vi "Main.vi"(8 "error in (no error)":T1) -> (0 "error out":T1)   [LabVIEW 2019, in "GUI.lvlib"]
uses:
  GUI.lvlib
  SubVIs/mmWave instrument_class/BurstMode.ctl
  SubVIs/mmWave instrument_class/RFConfig.ctl
  mmw_command_lib/src_LabVIEW/mmW_commands/TypeDefs/commands.ctl
  SubVIs/mmWave instrument_class/Instrument mode.ctl
  <vilib>/Utility/miscctls.llb/LVPointTypeDef.ctl
  SubVIs/mmWave data_class/mmWave data.lvclass
  SubVIs/Shared/Config state.ctl
  SubVIs/mmWave instrument_class/System info.ctl
  SubVIs/mmWave instrument_class/System state.ctl
  SubVIs/mmWave instrument_class/Instrument state.ctl
  SubVIs/mmWave instrument_class/Sync mode.ctl
  SubVIs/mmWave instrument_class/RF port info.ctl
  <vilib>/Utility/miscctls.llb/LVBoundsTypeDef.ctl
  SubVIs/Shared/CMD Configure RF.ctl
  SubVIs/Shared/CMD SetFS.ctl
  SubVIs/Shared/CMD Read RX index.ctl
  SubVIs/Shared/CMD Start.ctl
  SubVIs/Shared/CMD Trigger burst.ctl
  SubVIs/Shared/CMD Enable.ctl
  ee9e3aa9-1db0-42b0-80bd-b9c1fa160769.vi
  ce4761a1-2a1f-4738-b255-3cdb7d756e6c.vi
  SubVIs/IQBurst_memo_class/IQBurst_memo.lvclass
  C:/Barkhausen mmWave radar/Development/modules/mmw_instrument/src_LabVIEW/Host/SubVIs/mmWave data_class/mmWave data.lvclass
  SubVIs/Shared/Comm GV.vi
  SubVIs/Shared/System GV.vi
  HW Control/HW GV.vi
  Log/Log GV.vi
  <userlib>/_OpenG.lib/file/file.llb/Strip Path Extension - String__ogtk.vi
  <userlib>/_OpenG.lib/array/array.llb/Index 1D Array Elements (String)__ogtk.vi
  <vilib>/Utility/file.llb/Read Delimited Spreadsheet (string).vi
  Intertarget communication/UE_master_class/UE_master.lvclass
  Intertarget communication/NS master_class/NS master.lvclass
  SubVIs/Shared/Shared.lvlib
  HW Control/HW Control.lvlib
  Data Managment/DataManagment.lvlib
  SubVIs/mmWave instrument_class/mmWave instrument.lvclass
  <vilib>/addons/_JKI.lib/Serialization/JSON/JKI JSON Serialization.lvlib
  Log/Log.lvlib
  mmw_command_lib/src_LabVIEW/mmW_commands/mmW_commands.lvlib
  Intertarget communication/CommandResponse communication.lvlib
panel:
  out "TX records memory":dbl format="%#_6pB"
  out "RX records memory:":dbl format="%#_6pB"
  out "mode":string="RF"
  out "mmW class":string
  out "App version":string
  out "System ID":string
  out "Command resp":string
  in  "stop":bool
  in  "Console":enum32{"No Selection", "Config", "Control 2"}(radio)=enum."Config"
  in  "Control tab":enum32{"0", "1"}(tab)
  in  "RX Sampling frequency":dbl=3072000000.0 format="%#_6pHz"
  in  "TX Sampling frequency":dbl=3072000000.0 format="%#_6pHz"
  in  "RF.set fs":bool
  in  "RF.set":bool
  in  "RX":T2 {"Gain" format="%#_6fdb"; "Frequency" format="%#_6pHz"}
  in  "TX":T2 {"Gain" format="%#_6fdb"; "Frequency" format="%#_6pHz"}
  in  "Slave.LO share en":bool=TRUE caption="LO share"
  in  "Slave.Trig share en":bool=TRUE caption="Trigger share"
  in  "HW.Initialize":bool
  in  "EQ enable":bool caption="Checkbox"
  in  "EQ.Start":bool
  in  "Burst mode":T3
  in  "Acquisition duration":dbl=0.0008 format="%#_6ps"
  in  "HW.Stop":bool
  in  "HW.trig":bool
  in  "HW.Start":bool
  in  "HW.reset":bool
  in  "EQ.Stop":bool
  in  "HW.fetch":bool
  in  "init_mode":T4
  in  "DM.RX burst list":i32(listbox)
  in  "DM.Group":string(combo) caption="Burst group"
  in  "DM.clear":bool
  in  "DM.TX burst list":i32[](listbox)
  in  "DM.Add TX":bool
  out "Instrument status":string
  in  "Enable UI":bool=TRUE caption="Checkbox"
  in  "Display tab":T5(tab)
  in  "IQ.Plot":bool
  in  "IQ.Save":bool
  out "TX waveform":waveform(sgl)[](graph)
  out "RX waveform":waveform(sgl)[](graph)
  in  "Analysis.run":bool
  out "Analysis":cluster{"x0":dbl, "dx":dbl, "magnitude":dbl[]}[](graph)
  in  "Analysis.algo":string(combo)="Spectrum" caption="Algorithm"
  out "Analysis res":i32(listbox) caption="Results"
  in  "Log.reset":bool
  in  "Log tab":enum32{"Command log", "Timing", "Errors"}(tab)
  out "Debug.log":i32(listbox) caption="Command log"
  in  "Show all":bool=TRUE caption="Checkbox"
  in  "command filter":T6=enum."fetch"
  out "Execute start":dbl format="%#_6p"
  out "Execute trig":dbl format="%#_6p"
  out "Execute init":dbl format="%#_6p"
  out "Execute fetch":dbl format="%#_6p"
  out "Execute rf":dbl format="%#_6p"
  out "ZMQ command execution timing":cluster{"command":T6, "time":dbl}[](array[cluster]) {"time" format="%#_6ps"}
  out "Error history":T7(array[cluster])
  in  "HW.info":bool
  out "Sys info":string
  out "FIR coeff":dbl[][](graph)
  in  "EQ.plot":bool
  out "Channel response magnitude":cluster{"Ramp Pattern":dbl[], dbl[]}[](graph) caption="XY Graph - Dark"
  # "HW methods timing"
  # "Preview data from eq_coeff.csv and eq_channel.csv - output of last executed equalization"
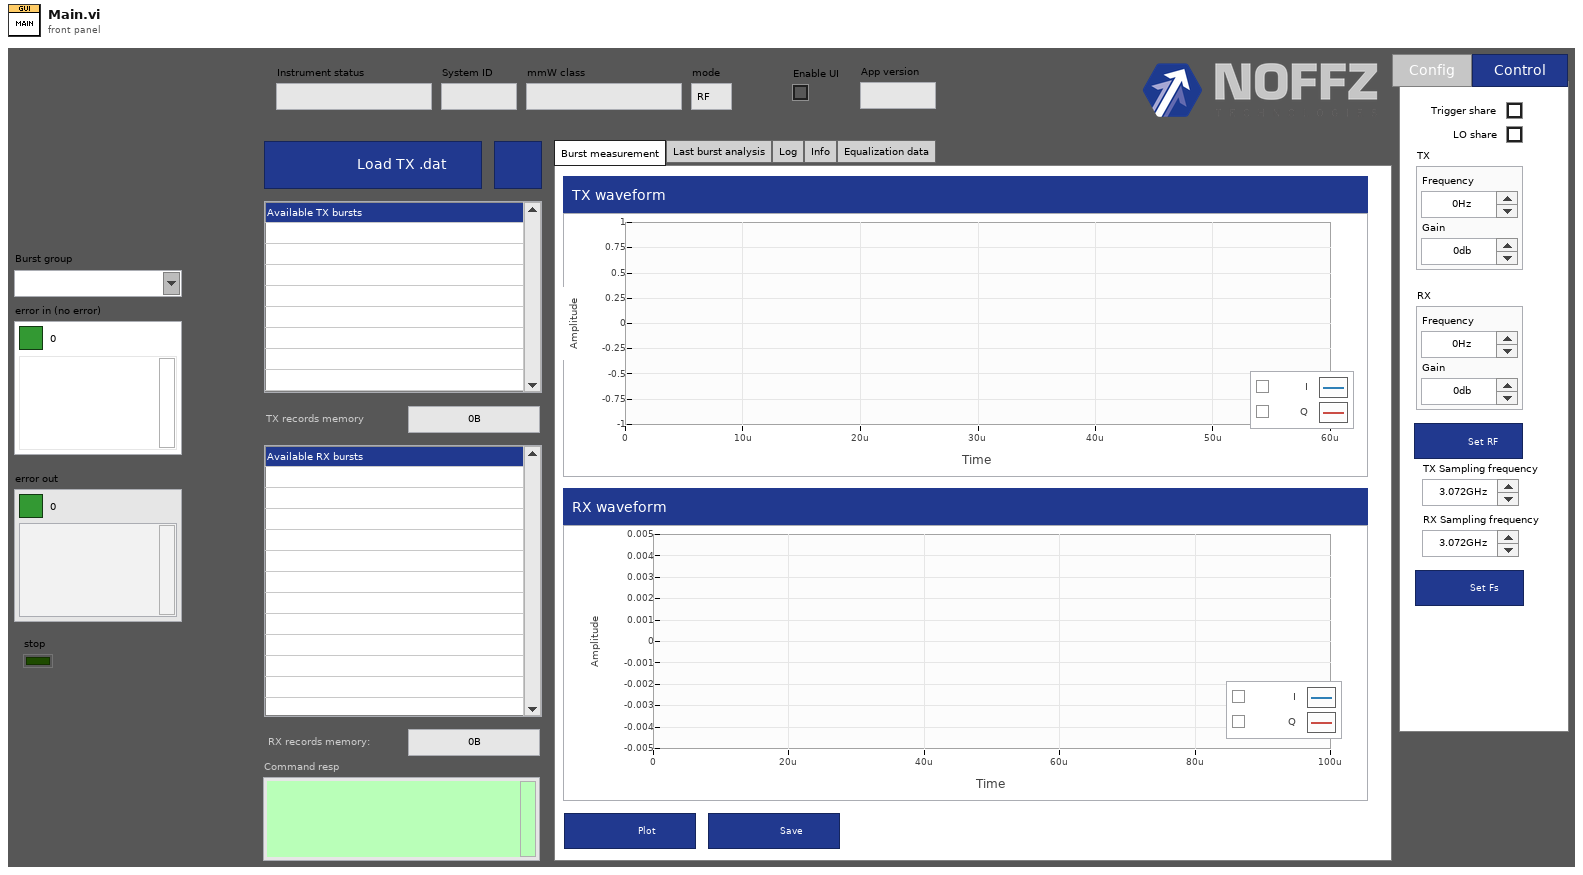
[diagram p1: front panel]
types:
  T1 = cluster{"Boolean Round":bool, "code":i32, "source":string}
  T2 = typedef "mmWave instrument.lvclass/RFConfig.ctl" = cluster{"Frequency":dbl, "Gain":dbl}
  T3 = typedef "mmWave instrument.lvclass/BurstMode.ctl" = enum16{"burst", "continuous"}
  T4 = typedef "mmWave instrument.lvclass/Instrument mode.ctl" = enum16{"RF", "IF", "BB"}
  T5 = enum32{"Burst measurement", "Last burst analysis", "Log", "Info", "Equalization data"}
  T6 = typedef "mmW_commands.lvlib/commands.ctl" = enum16{"configure_fs", "configure_rf", "configure_trigger", "equalization_enable", "equalization_start", "lo_sync_enable", "equalization_stop", "get_instrument_status", "get_versions", "initialize_hw", "pop_rx", "set_log_level", "Shutdown", "start", "start_instrument_app", "stop", "trans", "transceive", "trigger_burst", "trigger_sync_enable", "Write TX", "resp_generic", "resp_waveform", "send_trigger", "fetch", "transceive2"}
  T7 = cluster{"code":i32, "message":string, "source":string}[]
  T8 = enum32{"invalid app kind", "Development System", "Run Time System", "Student Edition", "Embedded LabVIEW", "Evaluation", "Custom"}
  T9 = cluster{"TX":refnum<class "mmWave data.lvclass">, "RX":refnum<class "mmWave data.lvclass">[]}
  T10 = typedef "LVPointTypeDef.ctl" = cluster{"Horizontal":i16, "Vertical":i16}
  T11 = typedef "LVBoundsTypeDef.ctl" = cluster{"Width":u32, "Height":u32}
  T12 = typedef "Shared.lvlib/CMD Configure RF.ctl" = cluster{"port":string, "fc":dbl, "gain":dbl}
  T13 = typedef "Shared.lvlib/CMD SetFS.ctl" = cluster{"port":string, "fs":dbl}
  T14 = enum16{"big-endian, network order", "native, host order", "little-endian"}
  T15 = typedef "Shared.lvlib/CMD Read RX index.ctl" = cluster{"burst index":i32}
  T16 = typedef "Shared.lvlib/CMD Start.ctl" = cluster{"Bursts":string[], "Acquisition duration":dbl}
  T17 = typedef "Shared.lvlib/CMD Trigger burst.ctl" = cluster{"Burst name":string, "Burst mode":T3}
  T18 = typedef "Shared.lvlib/CMD Enable.ctl" = cluster{"Enable":bool}
  T19 = cluster{"frequency offset (Hz)":dbl[], "response":cdb[]}
  T20 = enum32{"Burst measurement", "Last burst analysis", "Log", "Info"}
  T21 = typedef "Shared.lvlib/Config state.ctl" = cluster{"system info":T22, "state":T23, "tx":T26, "rx":T26, "versions":cluster{"app":string, "tx fpga":string, "rx fpga":string}}
  T22 = typedef "mmWave instrument.lvclass/System info.ctl" = cluster{"mmw instr":string, "max fs":dbl, "RX/LO1 src":string, "TX/LO1 src":string, "LO2 src":string, "RX LO1 export":bool, "TX LO1 export":bool, "LO2 export":bool, "TX LO1 export level":dbl, "RX LO1 export level":dbl, "LO2 export level":dbl}
  T23 = typedef "mmWave instrument.lvclass/System state.ctl" = cluster{"hw state":T24, "lo sync en":bool, "trig sync en":bool, "mode":T4, "sync":T25, "equalization en":bool}
  T24 = typedef "mmWave instrument.lvclass/Instrument state.ctl" = enum16{"Off", "Initialization", "Configuration", "Running", "Calibration"}
  T25 = typedef "mmWave instrument.lvclass/Sync mode.ctl" = enum16{"Slave", "Master"}
  T26 = typedef "mmWave instrument.lvclass/RF port info.ctl" = cluster{"fc":dbl, "gain":dbl, "fs":dbl, "trigger delay":dbl}
  T27 = typedef "DataManagment.lvlib/DM group info.ctl" = cluster{"group name":string, "burst names":string[], "burst sizes":dbl[], "Memory":dbl}
  T28 = typedef "CommandResponse communication.lvlib/Error response.ctl" = cluster{"code":i32, "message":string, "source":string}
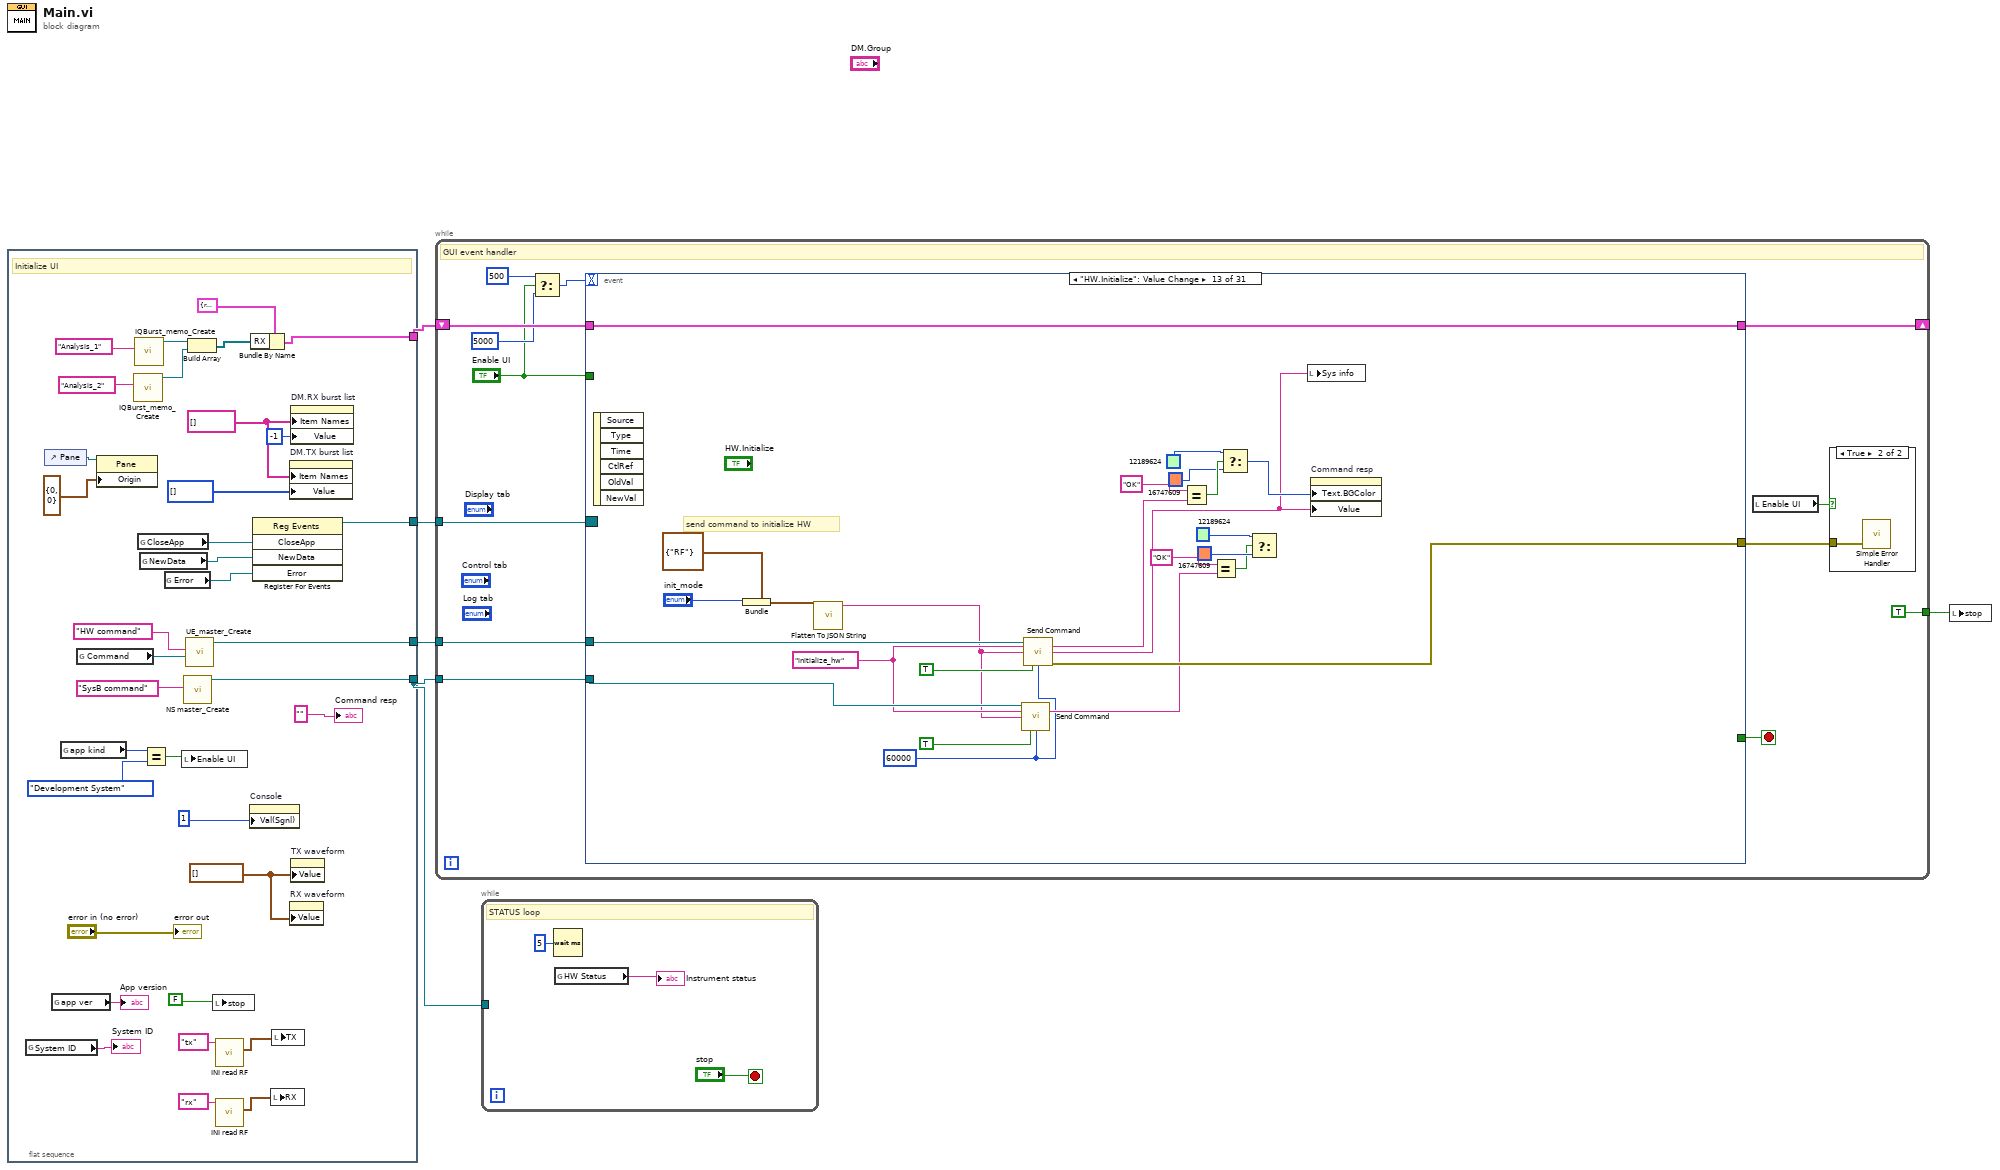
[diagram p0: block diagram]
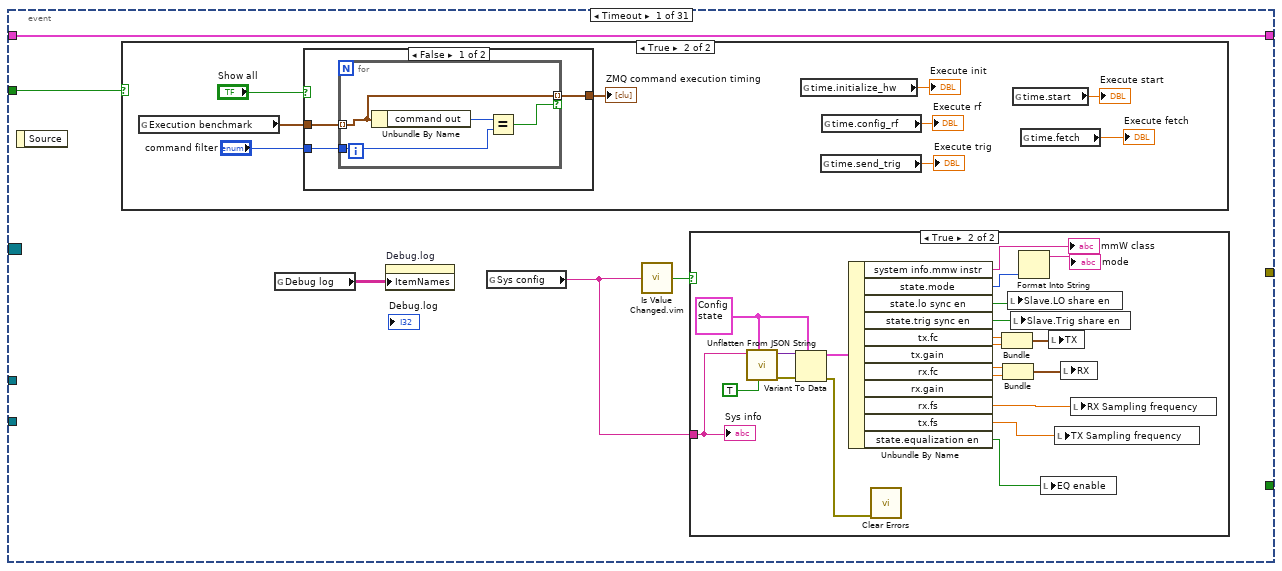
[diagram p3: hidden frame]
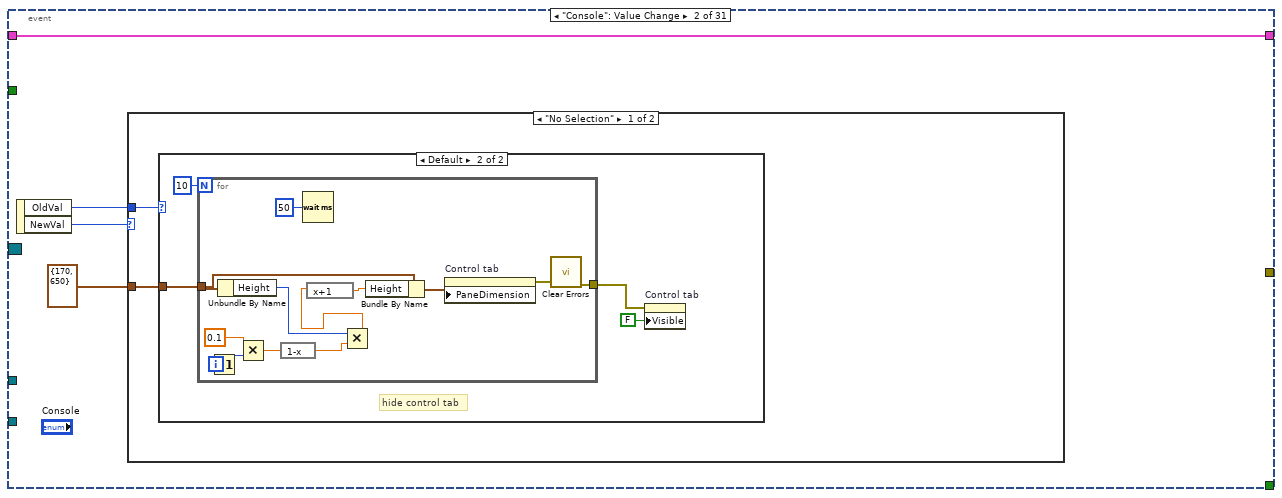
[diagram p7: hidden frame]
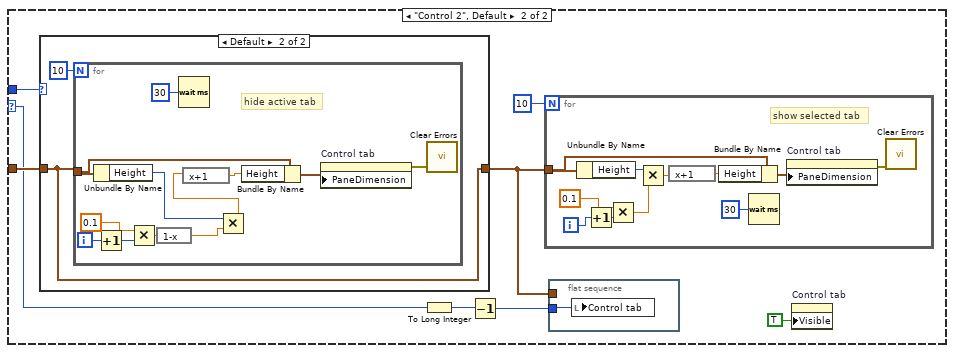
[diagram p9: hidden frame]
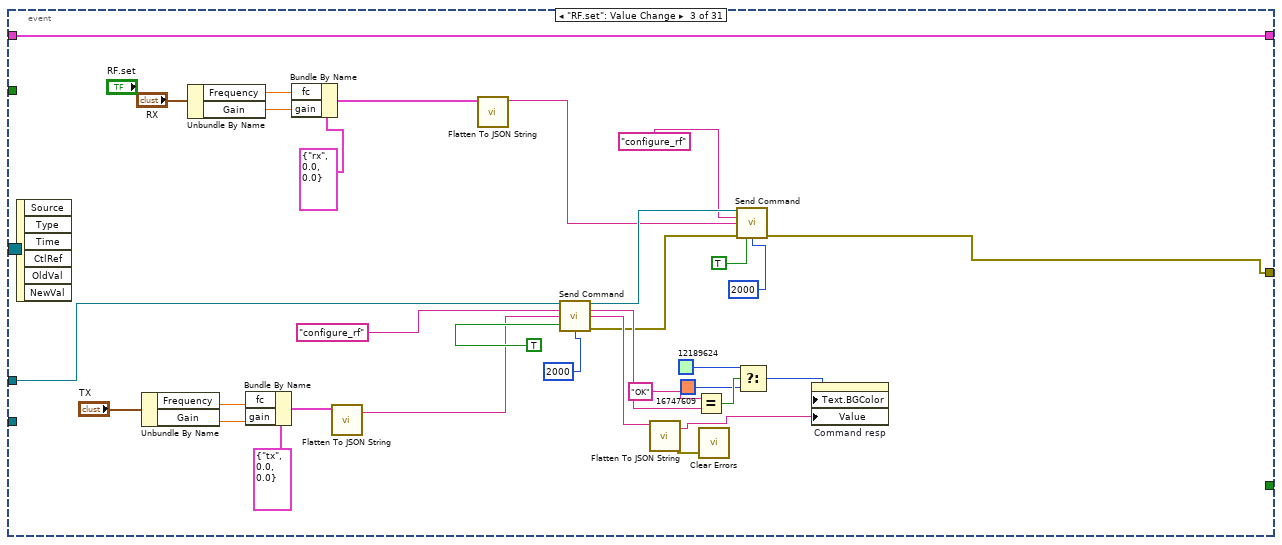
[diagram p11: hidden frame]
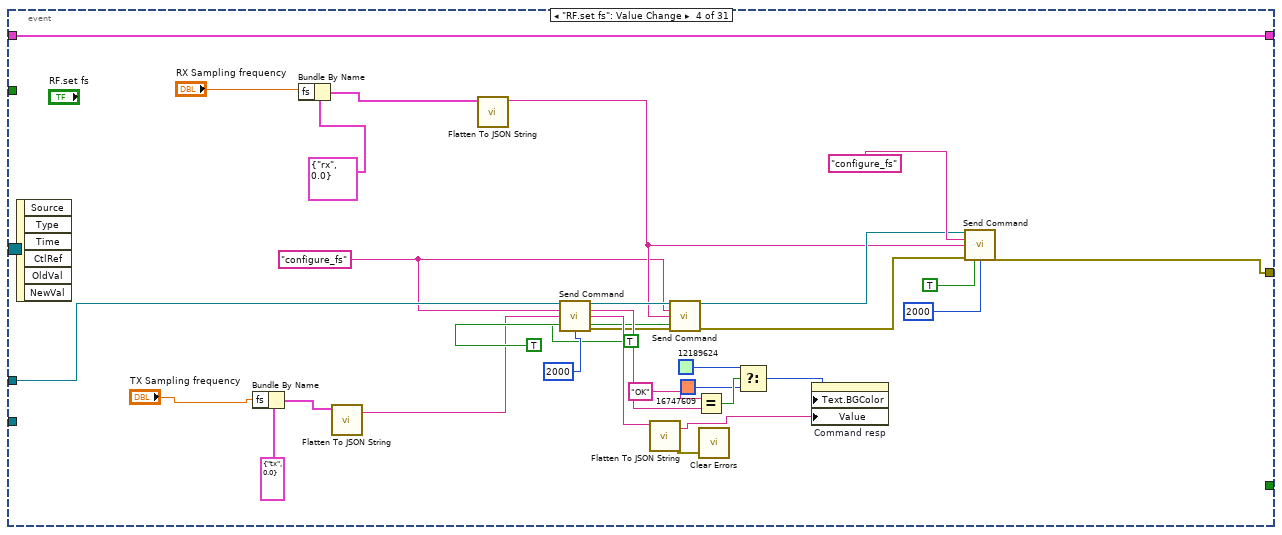
[diagram p12: hidden frame]
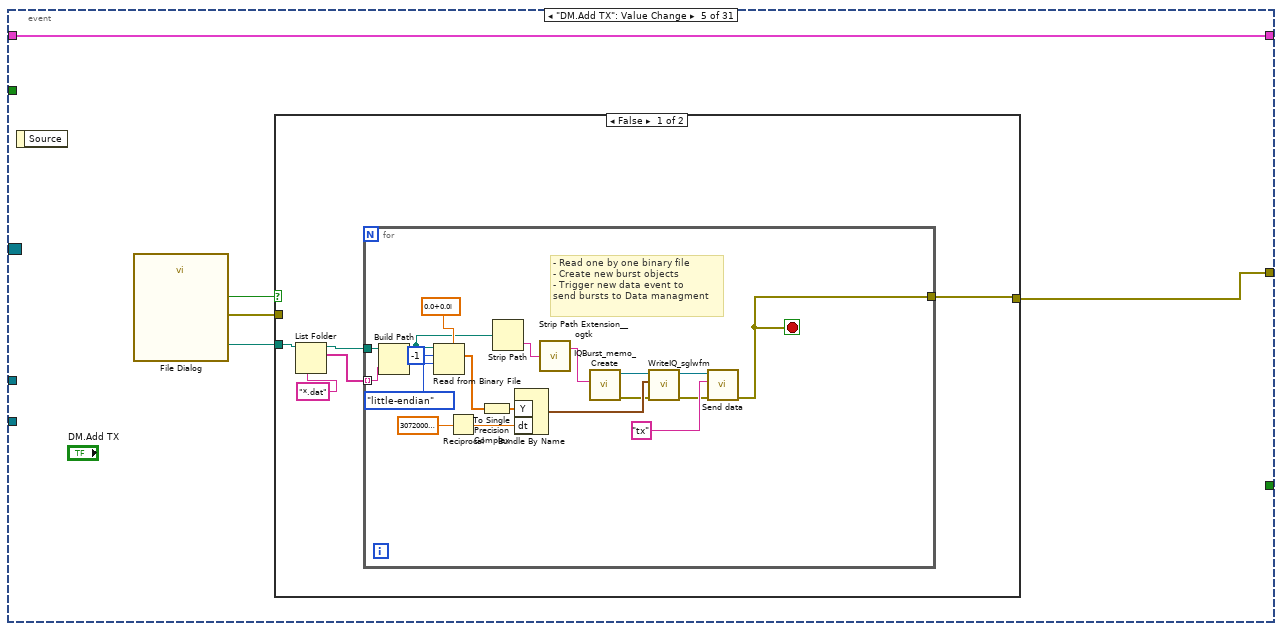
[diagram p13: hidden frame]
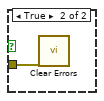
[diagram p14: hidden frame]
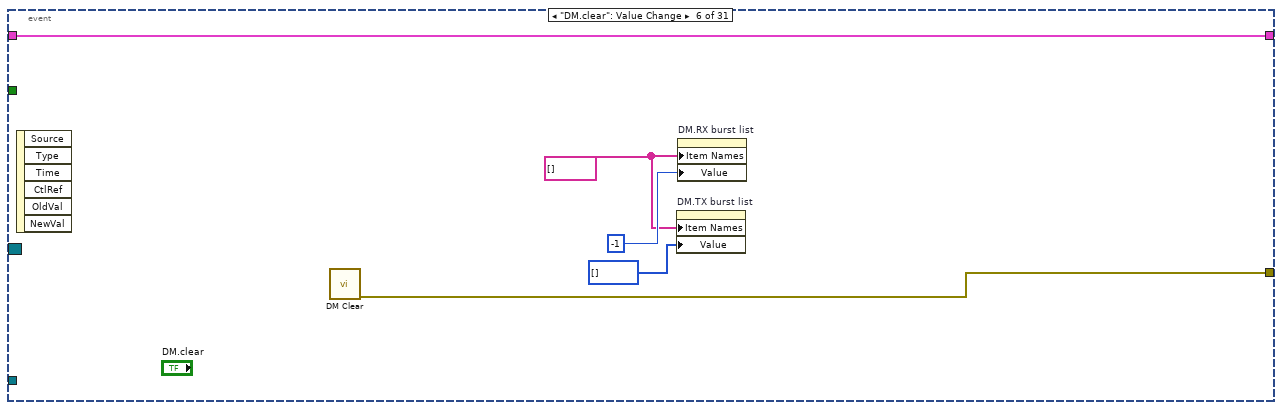
[diagram p15: hidden frame]
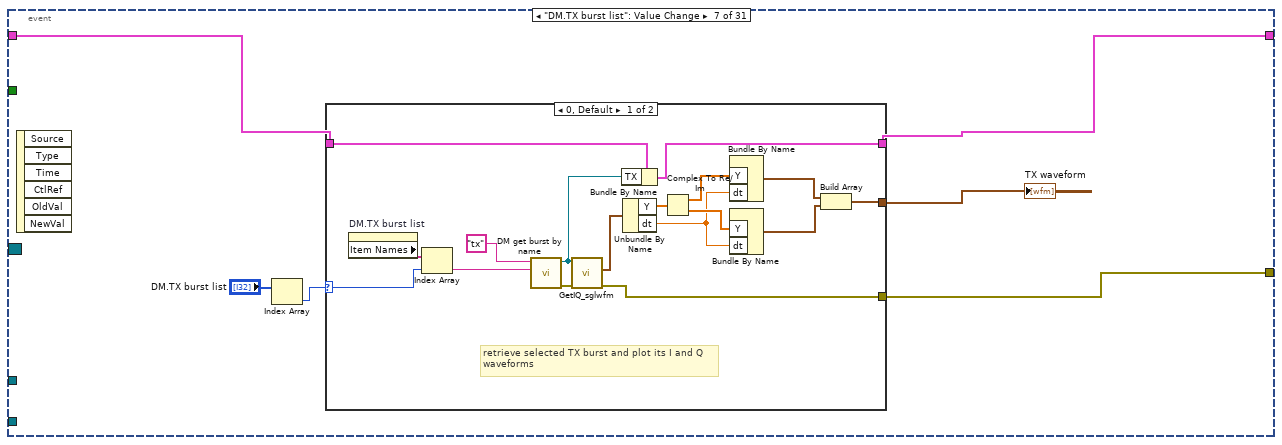
[diagram p16: hidden frame]
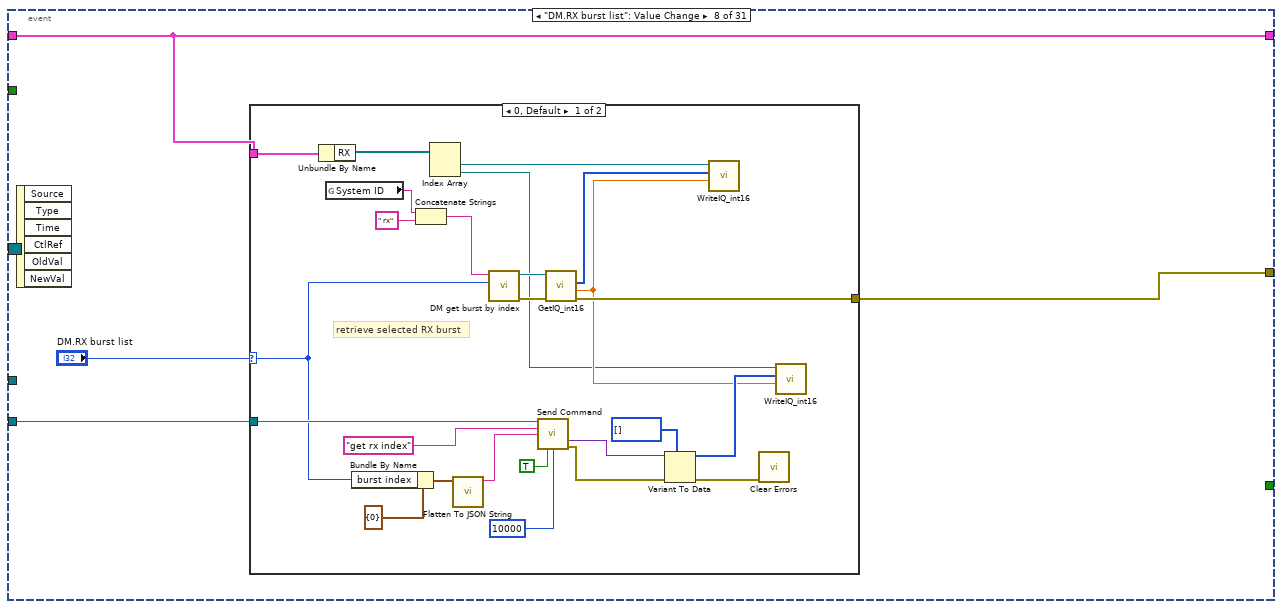
[diagram p18: hidden frame]
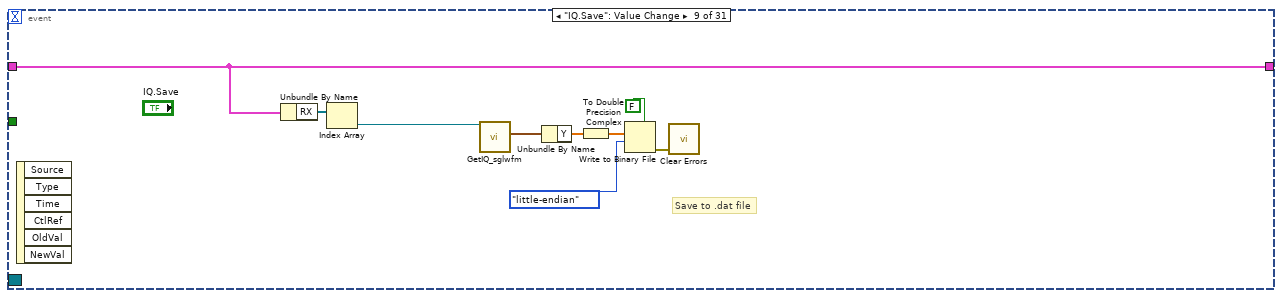
[diagram p20: hidden frame]
diagram:
  n1 = flat-sequence {
    tunnel: [w39] -> w5
    tunnel: [w28] -> w4
    tunnel: [w26] -> w2
    tunnel: [w17] -> w1
    frame #0 {
      w32 = waveform(sgl)[] [] ("RX waveform")
      w34 = string[] [] ("Item Names")
      # "Initialize UI"
      n2 = global read "System GV.vi" "System ID"() -> (→"System ID":string)
      n3 = control-ref of="Pane"() -> (w36:refnum<vi>)
      n4 = global read "System GV.vi" "app ver"() -> (→"App version":string)
      n5 = global read "System GV.vi" "app kind"() -> (w11:T8)
      n6 = global read "Comm GV.vi" "Command"() -> (w30:refnum<user-event>)
      n7 = property class="Pane"(reference=w36, "Origin"=T10 {"Horizontal"=0, "Vertical"=0}) -> ()  [unwired: 1 in, 2 out]
      n8 = call "IQBurst_memo_Create.vi"("burst name"="Analysis_2") -> ("reference out"=w20:refnum<class "IQBurst_memo.lvclass">)  [unwired: 9 in, 1 out]
      n9 = call "IQBurst_memo_Create.vi"("burst name"="Analysis_1") -> ("reference out"=w21:refnum<class "IQBurst_memo.lvclass">)  [unwired: 9 in, 1 out]
      n10 = global read "Comm GV.vi" "CloseApp"() -> (w40:refnum<user-event>)
      n11 = global read "Comm GV.vi" "NewData"() -> (w38:refnum<user-event>)
      n12 = Equal?(x=w11, y=T8."Development System") -> (x = y?=w9:bool)
      n13 = global read "Comm GV.vi" "Error"() -> (w37:refnum<user-event>)
      n14 = local write "Enable UI"(w9) -> ()
      n15 = call "NS master_Create.vi"("ID"="SysB command") -> ("reference out"=w26:refnum<class "NS master.lvclass">)  [unwired: 9 in, 1 out]
      n16 = call "UE_master_Create.vi"("Command UE"=w30, "ID"="HW command") -> ("reference out"=w28:refnum<class "UE_master.lvclass">)  [unwired: 8 in, 1 out]
      n17 = Build Array(w21, w20) -> (w18:refnum<class "IQBurst_memo.lvclass">[])
      n18 = local write "stop"(FALSE) -> ()
      n19 = call "INI read RF.vi"("Port"="tx") -> ("Config"=w15:T2)  [unwired: 8 in, 2 out]
      n20 = call "INI read RF.vi"("Port"="rx") -> ("Config"=w14:T2)  [unwired: 8 in, 2 out]
      n21 = property on="Console" class="RadioBtnsControl (strict)"("Val(Sgnl)"=1) -> ()  [unwired: 2 in, 2 out]
      n22 = Bundle By Name(cluster=T9 {"TX"=refnum, "RX"=[]} ("Cluster - Thin Border"), "RX"=w18) -> (w17:T9)
      n23 = register-events(w40, w38, w37) -> (reference out=w39:refnum<event-registration>)  [unwired: 2 in, 1 out]
      n24 = local write "RX"(w14) -> ()
      n25 = local write "TX"(w15) -> ()
      n26 = property on="DM.TX burst list" class="LstBox (strict)"("Item Names"=w34, "Value"=i32[] [] ("TX.bursts")) -> ()  [unwired: 2 in, 2 out]
      n27 = property on="RX waveform" class="WFGraph (strict)"("Value"=w32) -> ()  [unwired: 2 in, 2 out]
      n28 = property on="DM.RX burst list" class="LstBox (strict)"("Item Names"=w34, "Value"=-1 ("DM.RX burst list")) -> ()  [unwired: 2 in, 2 out]
      n29 = property on="TX waveform" class="WFGraph (strict)"("Value"=w32) -> ()  [unwired: 2 in, 2 out]
      "Command resp" <- "" ("HW response")
      "error out" <- "error in (no error)"
    }
  }
  n30 = while {
    tunnel: w5 -> [w53]
    tunnel: w4 -> [w50]
    tunnel: w2 -> [w49]
    tunnel: [TRUE] -> w3
    shift-right: [w46] -> _
    shift-left: w1 -> [w47]
    stop <- w52 stop-if-true
    # "GUI event handler"
    n31 = Select(t=500, s="Enable UI", f=5000) -> (s? t:f=w43:i32)
    n32 = event shown="[12] \"HW.Initialize\": Value Change" {
      selector: w53 -> [_ _ _ _ _ _ _ _ _ _ _ _ _ _ _ _ _ _ _ _ _ _ _ _ _ _ _ _ _ _ _]
      dyn-events: _ -> [_ _ _ _ _ _ _ _ _ _ _ _ _ _ _ _ _ _ _ _ _ _ _ _ _ _ _ _ _ _ _]
      timeout: w43 -> [_ _ _ _ _ _ _ _ _ _ _ _ _ _ _ _ _ _ _ _ _ _ _ _ _ _ _ _ _ _ _]
      tunnel: [_ _ _ _ _ _ _ _ _ _ _ _ _ _ _ _ _ _ _ _ _ _ _ _ _ TRUE _ _ _ w713 w715] -> w52
      tunnel: [_ _ w156 w197 w222 w253 w257 w281 _ _ w350 w370 w394 w427 w453 w482 w507 w531 w555 w583 _ w638 w666 _ w682 _ w698 _ _ w710 w717] -> w51
      tunnel: w50 -> [_ _ w175 w206 _ _ _ _ _ _ w351 w371 w395 w426 w451 w478 w505 w529 w553 w581 _ w636 w664 _ _ _ _ _ _ _ _]
      tunnel: w49 -> [_ _ _ _ _ _ _ w278 _ _ w349 w369 w393 w425 w450 w477 w504 w528 w552 w580 _ w635 w663 _ _ _ _ _ _ _ _]
      tunnel: w47 -> [w59 w98 w187 w218 w219 w250 w256 w279 w315 w318 w332 w353 w377 w400 w431 w454 w483 w509 w533 w561 w610 w616 w644 w671 w681 w689 w699 w705 w708 w709 w716]
      tunnel: [w59 w98 w187 w218 w219 w250 w255 w279 w315 w318 w332 w353 w377 w400 w431 w454 w483 w509 w533 w561 w610 w616 w644 w671 w681 w689 w699 w705 w708 w709 w716] -> w46
      tunnel: "Enable UI" -> [w58 _ _ _ _ _ _ _ _ _ _ _ _ _ _ _ _ _ _ _ _ _ _ _ _ _ _ _ _ _ _]
      event Timeout {
        n33 = event-data() -> ()  [unwired: 1 in, 1 out]
        n34 = case shown="True" w58 {
          frame False {
          }
          frame True {
            n35 = global read "Log GV.vi" "Execution benchmark"() -> (w89:cluster{"command out":T6, "final time":dbl}[])
            n36 = case shown="False" "Show all" {
              tunnel: w89 -> [w92 w97]
              tunnel: [w91 w97] -> w81
              tunnel: "command filter" -> [w90 _]
              frame False {
                n37 = for {
                  tunnel: w92 -> [w95] mode=indexing
                  tunnel: [w95] -> w91 mode=indexing if=w94
                  tunnel: w90 -> [w93]
                  n38 = Unbundle By Name(w95) -> ("command out"=w96:T6)
                  n39 = Equal?(x=w96, y=w93) -> (x = y?=w94:bool)
                }
              }
              frame True {
              }
            }
            "ZMQ command execution timing" <- w81
            n40 = global read "Log GV.vi" "time.initialize_hw"() -> (→"Execute init":dbl)
            n41 = global read "Log GV.vi" "time.send_trig"() -> (→"Execute trig":dbl)
            n42 = global read "Log GV.vi" "time.config_rf"() -> (→"Execute rf":dbl)
            n43 = global read "Log GV.vi" "time.start"() -> (→"Execute start":dbl)
            n44 = global read "Log GV.vi" "time.fetch"() -> (→"Execute fetch":dbl)
          }
        }
        n45 = global read "Log GV.vi" "Debug log"() -> (w57:string[][])
        n46 = property on="Debug.log" class="MCListbox (strict)"("ItemNames"=w57) -> ()  [unwired: 2 in, 2 out]
        n47 = global read "System GV.vi" "Sys config"() -> (w55:string)
        n48 = call "Is Value Changed.vim"("value"=w55) -> ("changed or first call?"=w56:bool)
        n49 = case shown="True" w56 {
          tunnel: w55 -> [_ w65]
          frame False {
          }
          frame True {
            w77 = T21 {"system info"={"mmw instr"="", "max fs"=0.0, "RX/LO1 src"="", "TX/LO1 src"="", "LO2 src"="", "RX LO1 export"=FALSE, "TX LO1 export"=FALSE, "LO2 export"=FALSE, "TX LO1 export level"=0.0, "RX LO1 export level"=0.0, "LO2 export level"=0.0}, "state"={"hw state"=enum."Off", "lo sync en"=FALSE, "trig sync en"=FALSE, "mode"=enum."RF", "sync"=enum."Slave", "equalization en"=FALSE}, "tx"={"fc"=0.0, "gain"=0.0, "fs"=0.0, "trigger delay"=0.0}, "rx"={"fc"=0.0, "gain"=0.0, "fs"=0.0, "trigger delay"=0.0}, "versions"={"app"="", "tx fpga"="", "rx fpga"=""}} ("Transciever config")
            n50 = call <vilib>:"Unflatten From JSON String.vi"("Nulls as Defaults (F)"=TRUE, "Type and Defaults"=w77, "JSON String"=w65) -> ("error out"=w80:errorcluster, "Variant"=w79:variant)  [unwired: 7 in]
            n51 = Variant To Data(error in=w80, type=w77, Variant=w79) -> (data=w66:T21, error out=w64:errorcluster)
            n52 = Unbundle By Name(w66) -> ("system info.mmw instr"=→"mmW class":string, "state.mode"=w60:T4, "state.lo sync en"=w75:bool, "state.trig sync en"=w76:bool, "tx.fc"=w74:dbl, "tx.gain"=w73:dbl, "rx.fc"=w70:dbl, "rx.gain"=w69:dbl, "rx.fs"=w68:dbl, "tx.fs"=w67:dbl, "state.equalization en"=w61:bool)
            n53 = call <vilib>:"Clear Errors.vi"("error in (no error)"=w64) -> ()  [unwired: 5 in, 2 out]
            n54 = Bundle("fc"=w74, "gain"=w73) -> (w72:cluster{"fc":dbl, "gain":dbl})  [unwired: 1 in]
            n55 = Bundle("fc"=w70, "gain"=w69) -> (w71:cluster{"fc":dbl, "gain":dbl})  [unwired: 1 in]
            n56 = local write "Slave.LO share en"(w75) -> ()
            n57 = local write "Slave.Trig share en"(w76) -> ()
            n58 = Format Into String(w60) -> (resulting string=→"mode":string)  [unwired: 3 in, 1 out]
            n59 = local write "EQ enable"(w61) -> ()
            n60 = local write "TX"(w72) -> ()
            n61 = local write "TX Sampling frequency"(w67) -> ()
            n62 = local write "RX"(w71) -> ()
            n63 = local write "RX Sampling frequency"(w68) -> ()
            "Sys info" <- w65
          }
        }
      }
      event "Console": Value Change {
        n64 = event-data() -> ("OldVal"=w100:enum32{"No Selection", "Config", "Control 2"}, "NewVal"=w101:enum32{"No Selection", "Config", "Control 2"})  [unwired: 1 in]
        n65 = case shown="\"No Selection\"" w101 {
          selector: w101 -> [_ w125]
          tunnel: T11 {"Width"=170, "Height"=650} ("Tab Control Pane Dimension") -> [w103 w128]
          tunnel: w100 -> [w102 w127]
          frame "No Selection" {
            n66 = case shown="Default" w102 {
              tunnel: w103 -> [_ w106]
              frame "No Selection" {
              }
              frame Default {
                # "hide control tab"
                n67 = for {
                  N: 10 -> [_]
                  tunnel: w106 -> [w116]
                  tunnel: [w108] -> w104
                  i -> [w119]
                  n68 = Increment(x=w119) -> (x+1=w109:i32)
                  n69 = Unbundle By Name(w116) -> ("Height"=w117:u32)
                  n70 = Multiply(x=0.1 ("y"), y=w109) -> (x*y=w112:dbl)
                  n71 = expression code="1-x"(w112) -> (w111:dbl)
                  n72 = Wait (ms)(milliseconds to wait=u32 50) -> ()  [unwired: 1 out]
                  n73 = Multiply(x=w117, y=w111) -> (x*y=w114:dbl)
                  n74 = expression code="x+1"(w114) -> (w113:dbl)
                  n75 = Bundle By Name(cluster=w116, "Height"=w113) -> (w115:T11)
                  n76 = property on="Control tab" class="TabCtl (strict)"("PaneDimension"=w115) -> (error out=w110:errorcluster)  [unwired: 2 in, 1 out]
                  n77 = call <vilib>:"Clear Errors.vi"("error in (no error)"=w110) -> ("error out"=w108:errorcluster)  [unwired: 5 in, 1 out]
                }
                n78 = property on="Control tab" class="TabCtl (strict)"(error in=w104, "Visible"=FALSE) -> ()  [unwired: 1 in, 2 out]
              }
            }
          }
          frame "Control 2", Default {
            n79 = case shown="Default" w127 {
              tunnel: w128 -> [w141 w142]
              tunnel: [w141 w142] -> w122
              frame "No Selection" {
              }
              frame Default {
                n80 = for {
                  N: 10 -> [_]
                  tunnel: w142 -> [w151]
                  i -> [w154]
                  # "hide active tab"
                  n81 = Unbundle By Name(w151) -> ("Height"=w152:u32)
                  n82 = Increment(x=w154) -> (x+1=w144:i32)
                  n83 = Multiply(x=0.1 ("y"), y=w144) -> (x*y=w147:dbl)
                  n84 = expression code="1-x"(w147) -> (w146:dbl)
                  n85 = Wait (ms)(milliseconds to wait=u32 30) -> ()  [unwired: 1 out]
                  n86 = Multiply(x=w152, y=w146) -> (x*y=w149:dbl)
                  n87 = expression code="x+1"(w149) -> (w148:dbl)
                  n88 = Bundle By Name(cluster=w151, "Height"=w148) -> (w150:T11)
                  n89 = property on="Control tab" class="TabCtl (strict)"("PaneDimension"=w150) -> (error out=w145:errorcluster)  [unwired: 2 in, 1 out]
                  n90 = call <vilib>:"Clear Errors.vi"("error in (no error)"=w145) -> ()  [unwired: 5 in, 2 out]
                }
              }
            }
            n91 = To Long Integer(number=w125) -> (32bit integer=w126:i32)
            n92 = Decrement(x=w126) -> (x-1=w124:i32)
            n93 = for {
              N: 10 -> [_]
              tunnel: w122 -> [w137]
              i -> [w133]
              # "show selected tab"
              n94 = Unbundle By Name(w137) -> ("Height"=w138:u32)
              n95 = Increment(x=w133) -> (x+1=w130:i32)
              n96 = Multiply(x=0.1 ("y"), y=w130) -> (x*y=w131:dbl)
              n97 = Multiply(x=w138, y=w131) -> (x*y=w136:dbl)
              n98 = expression code="x+1"(w136) -> (w132:dbl)
              n99 = Bundle By Name(cluster=w137, "Height"=w132) -> (w135:T11)
              n100 = Wait (ms)(milliseconds to wait=u32 30) -> ()  [unwired: 1 out]
              n101 = property on="Control tab" class="TabCtl (strict)"("PaneDimension"=w135) -> (error out=w134:errorcluster)  [unwired: 2 in, 1 out]
              n102 = call <vilib>:"Clear Errors.vi"("error in (no error)"=w134) -> ()  [unwired: 5 in, 2 out]
            }
            n103 = flat-sequence {
              tunnel: w124 -> [w129]
              tunnel: w122 -> [_]
              frame #0 {
                n104 = local write "Control tab"(w129) -> ()
              }
            }
            n105 = property on="Control tab" class="TabCtl (strict)"("Visible"=TRUE) -> ()  [unwired: 2 in, 2 out]
          }
        }
      }
      event "RF.set": Value Change {
        n106 = event-data() -> ()  [unwired: 1 in, 6 out]
        n107 = Unbundle By Name("TX") -> ("Frequency"=w171:dbl, "Gain"=w170:dbl)
        n108 = Unbundle By Name("RX") -> ("Frequency"=w163:dbl, "Gain"=w164:dbl)
        n109 = Bundle By Name(cluster=T12 {"port"="tx", "fc"=0.0, "gain"=0.0} ("Configure RF command"), "fc"=w171, "gain"=w170) -> (w169:T12)
        n110 = Bundle By Name(cluster=T12 {"port"="rx", "fc"=0.0, "gain"=0.0} ("Configure RF command"), "fc"=w163, "gain"=w164) -> (w165:T12)
        n111 = call <vilib>:"Flatten To JSON String.vi"("Variant"=w169) -> ("JSON String"=w168:string)  [unwired: 9 in, 1 out]
        n112 = call <vilib>:"Flatten To JSON String.vi"("Variant"=w165) -> ("JSON String"=w160:string)  [unwired: 9 in, 1 out]
        n113 = call-dynamic "Send Command.vi"("reference in"=w175, "message"="configure_rf", "parameters"=w168, "response?"=TRUE, "timeout"=2000) -> ("reference out"=w167:refnum<class "UE_master.lvclass">, "status"=w184:string, "reponse"=w182:string, "error out"=w157:errorcluster)  [unwired: 6 in, 1 out]
        n114 = call <vilib>:"Flatten To JSON String.vi"("Variant"=w182) -> ("error out"=w183:errorcluster, "JSON String"=w181:string)  [unwired: 9 in]
        n115 = Equal?(x="OK", y=w184) -> (x = y?=w186:bool)
        n116 = call <vilib>:"Clear Errors.vi"("error in (no error)"=w183) -> ()  [unwired: 5 in, 2 out]
        n117 = call-dynamic "Send Command.vi"("reference in"=w167, "message"="configure_rf", "parameters"=w160, "error in (no error)"=w157, "response?"=TRUE, "timeout"=2000) -> ("error out"=w156:errorcluster)  [unwired: 5 in, 4 out]
        n118 = Select(t=u32 12189624, s=w186, f=u32 16747609) -> (s? t:f=w185:u32)
        n119 = property on="Command resp" class="Str"("Text.BGColor"=w185, "Value"=w181) -> ()  [unwired: 2 in, 2 out]
      }
      event "RF.set fs": Value Change {
        w189 = "configure_fs" ("message")
        n120 = event-data() -> ()  [unwired: 1 in, 6 out]
        n121 = Bundle By Name(cluster=T13 {"port"="tx", "fs"=0.0} ("Set fs command"), "fs"="TX Sampling frequency") -> (w204:T13)
        n122 = Bundle By Name(cluster=T13 {"port"="rx", "fs"=0.0} ("Set fs command"), "fs"="RX Sampling frequency") -> (w201:T13)
        n123 = call <vilib>:"Flatten To JSON String.vi"("Variant"=w204) -> ("JSON String"=w203:string)  [unwired: 9 in, 1 out]
        n124 = call <vilib>:"Flatten To JSON String.vi"("Variant"=w201) -> ("JSON String"=w190:string)  [unwired: 9 in, 1 out]
        n125 = call-dynamic "Send Command.vi"("reference in"=w206, "message"=w189, "parameters"=w203, "response?"=TRUE, "timeout"=2000) -> ("reference out"=w194:refnum<class "UE_master.lvclass">, "status"=w215:string, "reponse"=w213:string, "error out"=w193:errorcluster)  [unwired: 6 in, 1 out]
        n126 = call <vilib>:"Flatten To JSON String.vi"("Variant"=w213) -> ("error out"=w214:errorcluster, "JSON String"=w212:string)  [unwired: 9 in]
        n127 = call-dynamic "Send Command.vi"("reference in"=w194, "message"=w189, "parameters"=w190, "error in (no error)"=w193, "response?"=TRUE) -> ("reference out"=w192:refnum<class "UE_master.lvclass">, "error out"=w191:errorcluster)  [unwired: 6 in, 3 out]
        n128 = Equal?(x="OK", y=w215) -> (x = y?=w217:bool)
        n129 = call <vilib>:"Clear Errors.vi"("error in (no error)"=w214) -> ()  [unwired: 5 in, 2 out]
        n130 = Select(t=u32 12189624, s=w217, f=u32 16747609) -> (s? t:f=w216:u32)
        n131 = property on="Command resp" class="Str"("Text.BGColor"=w216, "Value"=w212) -> ()  [unwired: 2 in, 2 out]
        n132 = call-dynamic "Send Command.vi"("reference in"=w192, "message"="configure_fs", "parameters"=w190, "error in (no error)"=w191, "response?"=TRUE, "timeout"=2000) -> ("error out"=w197:errorcluster)  [unwired: 5 in, 4 out]
      }
      event "DM.Add TX": Value Change {
        n133 = event-data() -> ()  [unwired: 1 in, 1 out]
        n134 = call "File Dialog"() -> ("selected path"=w221:path, "cancelled"=w223:bool, "error out"=w220:errorcluster)  [unwired: 12 in, 1 out]
        n135 = case shown="False" w223 {
          tunnel: [w224 _] -> w222
          tunnel: w221 -> [w228 _]
          tunnel: w220 -> [_ w248]
          frame False {
            n136 = List Folder(path=w228, pattern="*.dat" ("pattern (all files)")) -> (path out=w226:path, filenames=w225:string[])  [unwired: 2 in, 2 out]
            n137 = for {
              tunnel: [w238] -> w224
              tunnel: w226 -> [w244]
              tunnel: w225 -> [w243] mode=indexing
              stop <- w238 stop-if-true
              # "- Read one by one binary file\n- Create new burst objects\n- Trigger new data event to\nsend bursts to Data managment"
              n138 = Build Path(base path=w244, name or relative path=w243) -> (appended path=w242:path)
              n139 = Read from Binary File(5:cdb 0.0+0.0i ("TX.IQ signal"), 9:T14."little-endian" ("byte order (0:big-endian, network order)"), 10:-1 ("count (1)"), 11:w242) -> (2:w236:cdb[])  [unwired: 2 in, 3 out]
              n140 = Reciprocal(x=3072000000.0 ("sample rate (Hz)")) -> (1/x=w235:dbl)
              n141 = To Single Precision Complex(1:w236) -> (0:w232:csg[])
              n142 = Strip Path(path=w242) -> (name=w246:string)  [unwired: 1 out]
              n143 = Bundle By Name("Y"=w232, "dt"=w235) -> (w234:waveform(csg))  [unwired: 1 in]
              n144 = call-poly <userlib>:"Strip Path Extension__ogtk.vi"("path"=w246) -> ("root"=w245:string)  [unwired: 1 out]
              n145 = call "IQBurst_memo_Create.vi"("burst name"=w245) -> ("error out"=w233:errorcluster, "reference out"=w239:refnum<class "IQBurst_memo.lvclass">)  [unwired: 9 in]
              n146 = call-dynamic "WriteIQ_sglwfm.vi"("error in (no error)"=w233, "IQ wfm"=w234, "reference in"=w239) -> ("error out"=w231:errorcluster, "reference out"=w237:refnum<class "IQBurst_memo.lvclass">)  [unwired: 7 in]
              n147 = call "Send data.vi"("error in (no error)"=w231, "group"="tx", "Data"=w237) -> ("error out"=w238:T1)  [unwired: 8 in]
            }
          }
          frame True {
            n148 = call <vilib>:"Clear Errors.vi"("error in (no error)"=w248) -> ()  [unwired: 5 in, 2 out]
          }
        }
      }
      event "DM.clear": Value Change {
        w251 = string[] [] ("Item Names")
        n149 = event-data() -> ()  [unwired: 1 in, 6 out]
        n150 = call "DM Clear.vi"() -> ("error out"=w253:errorcluster)  [unwired: 11 in]
        n151 = property on="DM.TX burst list" class="LstBox (strict)"("Item Names"=w251, "Value"=i32[] [] ("DM.TX burst list")) -> ()  [unwired: 2 in, 2 out]
        n152 = property on="DM.RX burst list" class="LstBox (strict)"("Item Names"=w251, "Value"=-1 ("TX.bursts")) -> ()  [unwired: 2 in, 2 out]
      }
      event "DM.TX burst list": Value Change {
        n153 = event-data() -> ()  [unwired: 1 in, 6 out]
        n154 = Index Array(array="DM.TX burst list") -> (element=w254:i32)  [unwired: 1 in]
        n155 = case shown="0, Default" w254 {
          selector: w254 -> [w275 _]
          tunnel: [w264 _] -> w258
          tunnel: [w272 _] -> w257
          tunnel: w256 -> [w262 w277]
          tunnel: [w260 w277] -> w255
          frame 0, Default {
            # "retrieve selected TX burst and plot its I and Q\nwaveforms"
            n156 = property on="DM.TX burst list" class="LstBox (strict)"() -> ("Item Names"=w276:string[])  [unwired: 2 in, 2 out]
            n157 = Index Array(array=w276, index=w275) -> (element=w273:string)
            n158 = call "DM get burst by name.vi"("Burst name"=w273, "group"="tx") -> ("error out"=w274:errorcluster, "TX burst"=w261:refnum<class "mmWave data.lvclass">)  [unwired: 8 in]
            n159 = call-dynamic "GetIQ_sglwfm.vi"("error in (no error)"=w274, "reference in"=w261) -> ("error out"=w272:errorcluster, "IQ"=w263:waveform(csg))  [unwired: 7 in, 1 out]
            n160 = Bundle By Name(cluster=w262, "TX"=w261) -> (w260:T9)
            n161 = Unbundle By Name(w263) -> ("Y"=w270:csg[], "dt"=w265:dbl)
            n162 = Complex To Re/Im(x + iy=w270) -> (x=w269:sgl[], y=w267:sgl[])
            n163 = Bundle By Name("Y"=w269, "dt"=w265) -> (w268:waveform(sgl))  [unwired: 1 in]
            n164 = Bundle By Name("Y"=w267, "dt"=w265) -> (w266:waveform(sgl))  [unwired: 1 in]
            n165 = Build Array(w268, w266) -> (w264:waveform(sgl)[])
          }
          frame -1 {
          }
        }
        "TX waveform" <- w258
      }
      event "DM.RX burst list": Value Change {
        n166 = event-data() -> ()  [unwired: 1 in, 6 out]
        n167 = case shown="0, Default" "DM.RX burst list" {
          selector: "DM.RX burst list" -> [w292 _]
          tunnel: [w303 _] -> w281
          tunnel: w279 -> [w300 _]
          tunnel: w278 -> [w295 _]
          frame 0, Default {
            # "retrieve selected RX burst"
            n168 = Unbundle By Name(w300) -> ("RX"=w299:refnum<class "mmWave data.lvclass">[])
            n169 = global read "System GV.vi" "System ID"() -> (w301:string)
            n170 = Bundle By Name(cluster=T15 {"burst index"=0} ("read rx command"), "burst index"=w292) -> (w291:T15)
            n171 = Concatenate Strings(w301, " rx" ("group")) -> (w302:string)
            n172 = Index Array(array=w299) -> (element #1=w297:refnum<class "mmWave data.lvclass">, element #2=w285:refnum<class "mmWave data.lvclass">)  [unwired: 2 in]
            n173 = call <vilib>:"Flatten To JSON String.vi"("Variant"=w291) -> ("JSON String"=w290:string)  [unwired: 9 in, 1 out]
            n174 = call "DM get burst by index.vi"("Burst name"=w292, "group"=w302) -> ("error out"=w305:errorcluster, "TX burst"=w306:refnum<class "mmWave data.lvclass">)  [unwired: 8 in]
            n175 = call-dynamic "Send Command.vi"("reference in"=w295, "message"="get rx index", "parameters"=w290, "response?"=TRUE, "timeout"=10000) -> ("data"=w283:variant, "error out"=w284:errorcluster)  [unwired: 6 in, 3 out]
            n176 = call-dynamic "GetIQ_int16.vi"("error in (no error)"=w305, "reference in"=w306) -> ("error out"=w303:errorcluster, "dt"=w286:dbl, "data"=w298:i16[])  [unwired: 6 in, 1 out]
            n177 = Variant To Data(error in=w284, type=i16[] [], Variant=w283) -> (data=w287:i16[], error out=w288:errorcluster)
            n178 = call-dynamic "WriteIQ_int16.vi"("dt"=w286, "data"=w298, "reference in"=w297) -> ()  [unwired: 7 in, 2 out]
            n179 = call <vilib>:"Clear Errors.vi"("error in (no error)"=w288) -> ()  [unwired: 5 in, 2 out]
            n180 = call-dynamic "WriteIQ_int16.vi"("dt"=w286, "data"=w287, "reference in"=w285) -> ()  [unwired: 7 in, 2 out]
          }
          frame -1 {
          }
        }
      }
      event "IQ.Save": Value Change {
        # "Save to .dat file"
        n181 = event-data() -> ()  [unwired: 1 in, 6 out]
        n182 = Unbundle By Name(w315) -> ("RX"=w314:refnum<class "mmWave data.lvclass">[])
        n183 = Index Array(array=w314) -> (element=w313:refnum<class "mmWave data.lvclass">)  [unwired: 1 in]
        n184 = call-dynamic "GetIQ_sglwfm.vi"("reference in"=w313) -> ("IQ"=w312:waveform(csg))  [unwired: 8 in, 2 out]
        n185 = Unbundle By Name(w312) -> ("Y"=w311:csg[])
        n186 = To Double Precision Complex(1:w311) -> (0:w309:cdb[])
        n187 = Write to Binary File(data=w309, 5:FALSE ("prepend array or string size? (T)"), 9:T14."little-endian" ("byte order (0:big-endian, network order)")) -> (error out=w310:errorcluster)  [unwired: 3 in, 2 out]
        n188 = call <vilib>:"Clear Errors.vi"("error in (no error)"=w310) -> ()  [unwired: 5 in, 2 out]
      }
      event "IQ.Plot": Value Change {
        n189 = event-data() -> ()  [unwired: 1 in, 6 out]
        n190 = Unbundle By Name(w318) -> ("RX"=w317:refnum<class "mmWave data.lvclass">[])
        n191 = flat-sequence {
          tunnel: w317 -> [w319]
          tunnel: [w320] -> w316
          tunnel: w316 -> [w330]
          frame #0 {
            n192 = for {
              tunnel: [w323] -> w320 mode=concatenating
              tunnel: w319 -> [w321] mode=indexing
              n193 = call-dynamic "GetIQ_sglwfm.vi"("reference in"=w321) -> ("IQ"=w322:waveform(csg))  [unwired: 8 in, 2 out]
              n194 = Unbundle By Name(w322) -> ("Y"=w324:csg[], "dt"=w328:dbl)
              n195 = Complex To Re/Im(x + iy=w324) -> (x=w325:sgl[], y=w326:sgl[])
              n196 = Bundle By Name("Y"=w325, "dt"=w328) -> (w329:waveform(sgl))  [unwired: 1 in]
              n197 = Bundle By Name("Y"=w326, "dt"=w328) -> (w327:waveform(sgl))  [unwired: 1 in]
              n198 = Build Array(w329, w327) -> (w323:waveform(sgl)[])
            }
          }
          frame #1 {
            "RX waveform" <- w330
          }
          frame #2 {
            n199 = local write "IQ.Plot"(FALSE) -> ()
          }
        }
      }
      event "HW.reset": Value Change {
        w336 = 60000 ("timeout")
        w348 = "reset" ("message")
        # "send command to initialize HW"
        n200 = event-data() -> ()  [unwired: 1 in, 6 out]
        n201 = call-dynamic "Send Command.vi"("reference in"=w349, "message"=w348, "response?"=TRUE, "timeout"=w336) -> ("status"=w337:string)  [unwired: 7 in, 4 out]
        n202 = call-dynamic "Send Command.vi"("reference in"=w351, "message"=w348, "response?"=TRUE, "timeout"=w336) -> ("status"=w342:string, "reponse"=w335:string, "error out"=w350:errorcluster)  [unwired: 7 in, 2 out]
        n203 = Equal?(x="OK", y=w342) -> (x = y?=w347:bool)
        n204 = Equal?(x="OK", y=w337) -> (x = y?=w338:bool)
        n205 = Select(t=u32 12189624, s=w347, f=u32 16747609) -> (s? t:f=w346:u32)
        n206 = Select(t=u32 12189624, s=w338, f=u32 16747609) -> ()  [unwired: 1 out]
        n207 = property on="Command resp" class="Str"("Text.BGColor"=w346, "Value"=w335) -> ()  [unwired: 2 in, 2 out]
      }
      event "HW.info": Value Change {
        w356 = 60000 ("timeout")
        w368 = "get_config" ("message")
        # "send command to initialize HW"
        n208 = event-data() -> ()  [unwired: 1 in, 6 out]
        n209 = call-dynamic "Send Command.vi"("reference in"=w369, "message"=w368, "response?"=TRUE, "timeout"=w356) -> ("status"=w357:string)  [unwired: 7 in, 4 out]
        n210 = call-dynamic "Send Command.vi"("reference in"=w371, "message"=w368, "response?"=TRUE, "timeout"=w356) -> ("status"=w362:string, "reponse"=w352:string, "error out"=w370:errorcluster)  [unwired: 7 in, 2 out]
        n211 = Equal?(x="OK", y=w362) -> (x = y?=w367:bool)
        n212 = Equal?(x="OK", y=w357) -> (x = y?=w358:bool)
        n213 = Select(t=u32 12189624, s=w367, f=u32 16747609) -> (s? t:f=w366:u32)
        n214 = Select(t=u32 12189624, s=w358, f=u32 16747609) -> ()  [unwired: 1 out]
        n215 = local write "Sys info"(w352) -> ()
        n216 = property on="Command resp" class="Str"("Text.BGColor"=w366, "Value"=w352) -> ()  [unwired: 2 in, 2 out]
      }
      event "HW.Initialize": Value Change {
        w380 = 60000 ("timeout")
        w392 = "initialize_hw" ("message")
        # "send command to initialize HW"
        n217 = event-data() -> ()  [unwired: 1 in, 6 out]
        n218 = Bundle(cluster=cluster{"mode":T4} {"mode"=enum."RF"}, "mode"="init_mode") -> (w374:cluster{"mode":T4})
        n219 = call <vilib>:"Flatten To JSON String.vi"("Variant"=w374) -> ("JSON String"=w373:string)  [unwired: 9 in, 1 out]
        n220 = call-dynamic "Send Command.vi"("reference in"=w393, "message"=w392, "parameters"=w373, "response?"=TRUE, "timeout"=w380) -> ("status"=w381:string)  [unwired: 6 in, 4 out]
        n221 = call-dynamic "Send Command.vi"("reference in"=w395, "message"=w392, "parameters"=w373, "response?"=TRUE, "timeout"=w380) -> ("status"=w386:string, "reponse"=w376:string, "error out"=w394:errorcluster)  [unwired: 6 in, 2 out]
        n222 = Equal?(x="OK", y=w386) -> (x = y?=w391:bool)
        n223 = Equal?(x="OK", y=w381) -> (x = y?=w382:bool)
        n224 = Select(t=u32 12189624, s=w391, f=u32 16747609) -> (s? t:f=w390:u32)
        n225 = Select(t=u32 12189624, s=w382, f=u32 16747609) -> ()  [unwired: 1 out]
        n226 = local write "Sys info"(w376) -> ()
        n227 = property on="Command resp" class="Str"("Text.BGColor"=w390, "Value"=w376) -> ()  [unwired: 2 in, 2 out]
      }
      event "HW.Start": Value Change {
        w429 = "start" ("command")
        # "convert to ms"
        # "start operation:\n- load selected burst into instrument"
        n228 = event-data() -> ()  [unwired: 1 in, 6 out]
        n229 = property on="DM.TX burst list" class="LstBox (strict)"() -> ("Item Names"=w398:string[], "Value"=w397:i32[])  [unwired: 2 in, 2 out]
        n230 = call-poly <userlib>:"Index Array Elements__ogtk.vi"("indices"=w397, "array"=w398) -> ("elements"=w396:string[])  [unwired: 9 in]
        n231 = Bundle By Name(cluster=T16 {"Bursts"=[], "Acquisition duration"=0.0} ("Start command"), "Bursts"=w396, "Acquisition duration"="Acquisition duration") -> (w428:T16)
        n232 = Bundle By Name(cluster=T16 {"Bursts"=[], "Acquisition duration"=0.0} ("Start command"), "Bursts"=string[] [] ("TX bursts"), "Acquisition duration"="Acquisition duration") -> (w421:T16)
        n233 = call <vilib>:"Flatten To JSON String.vi"("Variant"=w428) -> ("JSON String"=w401:string)  [unwired: 9 in, 1 out]
        n234 = call <vilib>:"Flatten To JSON String.vi"("Variant"=w421) -> ("JSON String"=w402:string)  [unwired: 9 in, 1 out]
        n235 = call-dynamic "Send Command.vi"("reference in"=w425, "message"=w429, "parameters"=w402, "response?"=TRUE) -> ("status"=w409:string, "reponse"=w403:string)  [unwired: 7 in, 3 out]
        n236 = call-dynamic "Send Command.vi"("reference in"=w426, "message"=w429, "parameters"=w401, "response?"=TRUE, "timeout"=2000) -> ("status"=w410:string, "reponse"=w406:string, "error out"=w427:errorcluster)  [unwired: 6 in, 2 out]
        n237 = call <vilib>:"Flatten To JSON String.vi"("Variant"=w403) -> ("error out"=w404:errorcluster)  [unwired: 9 in, 1 out]
        n238 = call <vilib>:"Clear Errors.vi"("error in (no error)"=w404) -> ()  [unwired: 5 in, 2 out]
        n239 = call <vilib>:"Flatten To JSON String.vi"("Variant"=w406) -> ("error out"=w407:errorcluster, "JSON String"=w405:string)  [unwired: 9 in]
        n240 = Equal?(x="OK", y=w410) -> (x = y?=w419:bool)
        n241 = call <vilib>:"Clear Errors.vi"("error in (no error)"=w407) -> ()  [unwired: 5 in, 2 out]
        n242 = Equal?(x="OK", y=w409) -> (x = y?=w417:bool)
        n243 = Select(t=u32 12189624, s=w419, f=u32 16747609) -> (s? t:f=w418:u32)
        n244 = Select(t=u32 12189624, s=w417, f=u32 16747609) -> ()  [unwired: 1 out]
        n245 = property on="Command resp" class="Str"("Text.BGColor"=w418, "Value"=w405) -> ()  [unwired: 2 in, 2 out]
      }
      event "HW.Stop": Value Change {
        w452 = "stop" ("command")
        n246 = event-data() -> ()  [unwired: 1 in, 6 out]
        n247 = call-dynamic "Send Command.vi"("reference in"=w451, "message"=w452, "response?"=TRUE) -> ("status"=w439:string, "reponse"=w436:string, "error out"=w453:errorcluster)  [unwired: 8 in, 2 out]
        n248 = call-dynamic "Send Command.vi"("reference in"=w450, "message"=w452, "response?"=TRUE) -> ("status"=w438:string, "reponse"=w433:string)  [unwired: 8 in, 3 out]
        n249 = call <vilib>:"Flatten To JSON String.vi"("Variant"=w436) -> ("error out"=w434:errorcluster, "JSON String"=w435:string)  [unwired: 9 in]
        n250 = call <vilib>:"Flatten To JSON String.vi"("Variant"=w433) -> ("error out"=w432:errorcluster)  [unwired: 9 in, 1 out]
        n251 = call <vilib>:"Clear Errors.vi"("error in (no error)"=w434) -> ()  [unwired: 5 in, 2 out]
        n252 = call <vilib>:"Clear Errors.vi"("error in (no error)"=w432) -> ()  [unwired: 5 in, 2 out]
        n253 = Equal?(x="OK", y=w439) -> (x = y?=w448:bool)
        n254 = Equal?(x="OK", y=w438) -> (x = y?=w446:bool)
        n255 = Select(t=u32 12189624, s=w448, f=u32 16747609) -> (s? t:f=w447:u32)
        n256 = Select(t=u32 12189624, s=w446, f=u32 16747609) -> ()  [unwired: 1 out]
        n257 = property on="Command resp" class="Str"("Text.BGColor"=w447, "Value"=w435) -> ()  [unwired: 2 in, 2 out]
      }
      event "HW.trig": Value Change {
        w481 = "send_trigger" ("command")
        # "trigger single burst"
        n258 = event-data() -> ()  [unwired: 1 in, 6 out]
        n259 = Bundle By Name(cluster=T17 {"Burst name"="", "Burst mode"=enum."burst"} ("Trigger burst command"), "Burst mode"="Burst mode") -> (w473:T17)
        n260 = call <vilib>:"Flatten To JSON String.vi"("Variant"=w473) -> ("JSON String"=w455:string)  [unwired: 9 in, 1 out]
        n261 = call-dynamic "Send Command.vi"("reference in"=w478, "message"=w481, "parameters"=w455, "response?"=TRUE) -> ("status"=w463:string, "reponse"=w459:string, "error out"=w476:errorcluster)  [unwired: 7 in, 2 out]
        n262 = call-dynamic "Send Command.vi"("reference in"=w477, "message"=w481, "parameters"=w455, "response?"=TRUE) -> ("status"=w462:string, "reponse"=w456:string, "error out"=w475:errorcluster)  [unwired: 7 in, 2 out]
        n263 = call <vilib>:"Flatten To JSON String.vi"("Variant"=w459) -> ("error out"=w460:errorcluster, "JSON String"=w458:string)  [unwired: 9 in]
        n264 = Merge Errors(w476, w475) -> (w482:errorcluster)
        n265 = Equal?(x="OK", y=w463) -> (x = y?=w472:bool)
        n266 = Equal?(x="OK", y=w462) -> (x = y?=w470:bool)
        n267 = call <vilib>:"Flatten To JSON String.vi"("Variant"=w456) -> ("error out"=w457:errorcluster)  [unwired: 9 in, 1 out]
        n268 = Select(t=u32 12189624, s=w472, f=u32 16747609) -> (s? t:f=w471:u32)
        n269 = Select(t=u32 12189624, s=w470, f=u32 16747609) -> ()  [unwired: 1 out]
        n270 = call <vilib>:"Clear Errors.vi"("error in (no error)"=w457) -> ()  [unwired: 5 in, 2 out]
        n271 = call <vilib>:"Clear Errors.vi"("error in (no error)"=w460) -> ()  [unwired: 5 in, 2 out]
        n272 = property on="Command resp" class="Str"("Text.BGColor"=w471, "Value"=w458) -> ()  [unwired: 2 in, 2 out]
      }
      event "HW.fetch": Value Change {
        w506 = "fetch" ("command")
        # "trigger single burst"
        n273 = event-data() -> ()  [unwired: 1 in, 6 out]
        n274 = call-dynamic "Send Command.vi"("reference in"=w505, "message"=w506, "response?"=TRUE) -> ("status"=w491:string, "reponse"=w487:string, "error out"=w503:errorcluster)  [unwired: 8 in, 2 out]
        n275 = call-dynamic "Send Command.vi"("reference in"=w504, "message"=w506, "response?"=TRUE) -> ("status"=w490:string, "reponse"=w484:string, "error out"=w502:errorcluster)  [unwired: 8 in, 2 out]
        n276 = call <vilib>:"Flatten To JSON String.vi"("Variant"=w487) -> ("error out"=w488:errorcluster, "JSON String"=w486:string)  [unwired: 9 in]
        n277 = Merge Errors(w503, w502) -> (w507:errorcluster)
        n278 = Equal?(x="OK", y=w491) -> (x = y?=w500:bool)
        n279 = Equal?(x="OK", y=w490) -> (x = y?=w498:bool)
        n280 = call <vilib>:"Flatten To JSON String.vi"("Variant"=w484) -> ("error out"=w485:errorcluster)  [unwired: 9 in, 1 out]
        n281 = Select(t=u32 12189624, s=w500, f=u32 16747609) -> (s? t:f=w499:u32)
        n282 = Select(t=u32 12189624, s=w498, f=u32 16747609) -> ()  [unwired: 1 out]
        n283 = call <vilib>:"Clear Errors.vi"("error in (no error)"=w485) -> ()  [unwired: 5 in, 2 out]
        n284 = call <vilib>:"Clear Errors.vi"("error in (no error)"=w488) -> ()  [unwired: 5 in, 2 out]
        n285 = property on="Command resp" class="Str"("Text.BGColor"=w499, "Value"=w486) -> ()  [unwired: 2 in, 2 out]
      }
      event "EQ.Start": Value Change {
        w530 = "equalization_start" ("command")
        n286 = event-data() -> ()  [unwired: 1 in, 6 out]
        n287 = call-dynamic "Send Command.vi"("reference in"=w529, "message"=w530, "response?"=TRUE, "timeout"=5000) -> ("status"=w517:string, "reponse"=w514:string, "error out"=w531:errorcluster)  [unwired: 7 in, 2 out]
        n288 = call-dynamic "Send Command.vi"("reference in"=w528, "message"=w530, "response?"=TRUE) -> ("status"=w516:string, "reponse"=w511:string)  [unwired: 8 in, 3 out]
        n289 = call <vilib>:"Flatten To JSON String.vi"("Variant"=w514) -> ("error out"=w512:errorcluster, "JSON String"=w513:string)  [unwired: 9 in]
        n290 = call <vilib>:"Flatten To JSON String.vi"("Variant"=w511) -> ("error out"=w510:errorcluster)  [unwired: 9 in, 1 out]
        n291 = call <vilib>:"Clear Errors.vi"("error in (no error)"=w512) -> ()  [unwired: 5 in, 2 out]
        n292 = call <vilib>:"Clear Errors.vi"("error in (no error)"=w510) -> ()  [unwired: 5 in, 2 out]
        n293 = Equal?(x="OK", y=w517) -> (x = y?=w526:bool)
        n294 = Equal?(x="OK", y=w516) -> (x = y?=w524:bool)
        n295 = Select(t=u32 12189624, s=w526, f=u32 16747609) -> (s? t:f=w525:u32)
        n296 = Select(t=u32 12189624, s=w524, f=u32 16747609) -> ()  [unwired: 1 out]
        n297 = property on="Command resp" class="Str"("Text.BGColor"=w525, "Value"=w513) -> ()  [unwired: 2 in, 2 out]
      }
      event "EQ.Stop": Value Change {
        w554 = "equalization_stop" ("command")
        n298 = event-data() -> ()  [unwired: 1 in, 6 out]
        n299 = call-dynamic "Send Command.vi"("reference in"=w553, "message"=w554, "response?"=TRUE, "timeout"=5000) -> ("status"=w541:string, "reponse"=w538:string, "error out"=w555:errorcluster)  [unwired: 7 in, 2 out]
        n300 = call-dynamic "Send Command.vi"("reference in"=w552, "message"=w554, "response?"=TRUE) -> ("status"=w540:string, "reponse"=w535:string)  [unwired: 8 in, 3 out]
        n301 = call <vilib>:"Flatten To JSON String.vi"("Variant"=w538) -> ("error out"=w536:errorcluster, "JSON String"=w537:string)  [unwired: 9 in]
        n302 = call <vilib>:"Flatten To JSON String.vi"("Variant"=w535) -> ("error out"=w534:errorcluster)  [unwired: 9 in, 1 out]
        n303 = call <vilib>:"Clear Errors.vi"("error in (no error)"=w536) -> ()  [unwired: 5 in, 2 out]
        n304 = call <vilib>:"Clear Errors.vi"("error in (no error)"=w534) -> ()  [unwired: 5 in, 2 out]
        n305 = Equal?(x="OK", y=w541) -> (x = y?=w550:bool)
        n306 = Equal?(x="OK", y=w540) -> (x = y?=w548:bool)
        n307 = Select(t=u32 12189624, s=w550, f=u32 16747609) -> (s? t:f=w549:u32)
        n308 = Select(t=u32 12189624, s=w548, f=u32 16747609) -> ()  [unwired: 1 out]
        n309 = property on="Command resp" class="Str"("Text.BGColor"=w549, "Value"=w537) -> ()  [unwired: 2 in, 2 out]
      }
      event "EQ enable": Value Change {
        w582 = "equalization_enable" ("command")
        n310 = event-data() -> ()  [unwired: 1 in, 6 out]
        n311 = Bundle By Name(cluster=T18 {"Enable"=FALSE} ("Equalization command"), "Enable"="EQ enable") -> (w557:T18)
        n312 = Flatten To JSON(anything=w557) -> (JSON string=w556:string)  [unwired: 2 in, 1 out]
        n313 = call-dynamic "Send Command.vi"("reference in"=w581, "message"=w582, "parameters"=w556, "response?"=TRUE, "timeout"=5000) -> ("status"=w569:string, "reponse"=w566:string, "error out"=w583:errorcluster)  [unwired: 6 in, 2 out]
        n314 = call-dynamic "Send Command.vi"("reference in"=w580, "message"=w582, "parameters"=w556, "response?"=TRUE) -> ("status"=w568:string, "reponse"=w563:string)  [unwired: 7 in, 3 out]
        n315 = call <vilib>:"Flatten To JSON String.vi"("Variant"=w566) -> ("error out"=w564:errorcluster, "JSON String"=w565:string)  [unwired: 9 in]
        n316 = call <vilib>:"Flatten To JSON String.vi"("Variant"=w563) -> ("error out"=w562:errorcluster)  [unwired: 9 in, 1 out]
        n317 = call <vilib>:"Clear Errors.vi"("error in (no error)"=w564) -> ()  [unwired: 5 in, 2 out]
        n318 = call <vilib>:"Clear Errors.vi"("error in (no error)"=w562) -> ()  [unwired: 5 in, 2 out]
        n319 = Equal?(x="OK", y=w569) -> (x = y?=w578:bool)
        n320 = Equal?(x="OK", y=w568) -> (x = y?=w576:bool)
        n321 = Select(t=u32 12189624, s=w578, f=u32 16747609) -> (s? t:f=w577:u32)
        n322 = Select(t=u32 12189624, s=w576, f=u32 16747609) -> ()  [unwired: 1 out]
        n323 = property on="Command resp" class="Str"("Text.BGColor"=w577, "Value"=w565) -> ()  [unwired: 2 in, 2 out]
      }
      event "EQ.plot": Value Change {
        n324 = event-data() -> ()  [unwired: 1 in, 6 out]
        n325 = global read "System GV.vi" "mmw_instr app data"() -> (w607:path)
        n326 = Build Path(base path=w607, name or relative path="eq_channel.csv") -> (appended path=w598:path)
        n327 = Build Path(base path=w607, name or relative path="eq_coeff.csv") -> (appended path=w606:path)
        n328 = call "Load FIR coeff from CSV.vi"("Path"=w606) -> ("1D Array"=w605:cdb[])  [unwired: 8 in, 2 out]
        n329 = call-poly <vilib>:"Read Delimited Spreadsheet.vi"("file path (dialog if empty)"=w598, "delimiter (\\t)"="," ("delimiter (\\t)")) -> ("all rows"=w597:string[][])  [unwired: 8 in, 5 out]
        n330 = Complex To Re/Im(x + iy=w605) -> (x=w604:dbl[], y=w603:dbl[])
        n331 = Delete From Array(array=w597, index (row)=0) -> (array with subset deleted=w594:string[][])  [unwired: 2 in, 1 out]
        n332 = Build Array(w604, w603) -> (→"FIR coeff":dbl[][])
        n333 = Fract/Exp String To Number(string=w594) -> (number=w592:dbl[][])  [unwired: 3 in, 1 out]
        n334 = Index Array(array=w592, index (col) #1=0 ("disabled index (col)"), index (col) #2=1 ("disabled index (col)"), index (col) #3=2 ("disabled index (col)")) -> (element #1=w593:dbl[], element #2=w586:dbl[], element #3=w585:dbl[])  [unwired: 3 in]
        n335 = Polar To Complex(1:w585, 2:w586) -> (0:w584:cdb[])
        n336 = Bundle By Name(cluster=T19 {"frequency offset (Hz)"=[], "response"=[]} ("channel"), "frequency offset (Hz)"=w593, "response"=w584) -> (w587:T19)
        n337 = call "Calculate equalization FIR.vi"("channel"=w587, "FIR taps"=32, "Max FIR gain"=6.0) -> ("Mag response"=→"Channel response magnitude":cluster{"xi used":dbl[], "yi":dbl[]}[])  [unwired: 10 in, 2 out]
      }
      event "Slave.Trig share en": Value Change {
        w637 = "trig_share_enable" ("command")
        n338 = event-data() -> ()  [unwired: 1 in, 6 out]
        n339 = Bundle By Name(cluster=T18 {"Enable"=FALSE} ("Equalization command"), "Enable"="Slave.Trig share en") -> (w613:T18)
        n340 = Flatten To JSON(anything=w613) -> (JSON string=w612:string)  [unwired: 2 in, 1 out]
        n341 = call-dynamic "Send Command.vi"("reference in"=w636, "message"=w637, "parameters"=w612, "response?"=TRUE, "timeout"=5000) -> ("status"=w624:string, "reponse"=w621:string, "error out"=w638:errorcluster)  [unwired: 6 in, 2 out]
        n342 = call-dynamic "Send Command.vi"("reference in"=w635, "message"=w637, "parameters"=w612, "response?"=TRUE) -> ("status"=w623:string, "reponse"=w618:string)  [unwired: 7 in, 3 out]
        n343 = call <vilib>:"Flatten To JSON String.vi"("Variant"=w621) -> ("error out"=w619:errorcluster, "JSON String"=w620:string)  [unwired: 9 in]
        n344 = call <vilib>:"Flatten To JSON String.vi"("Variant"=w618) -> ("error out"=w617:errorcluster)  [unwired: 9 in, 1 out]
        n345 = call <vilib>:"Clear Errors.vi"("error in (no error)"=w619) -> ()  [unwired: 5 in, 2 out]
        n346 = call <vilib>:"Clear Errors.vi"("error in (no error)"=w617) -> ()  [unwired: 5 in, 2 out]
        n347 = Equal?(x="OK", y=w624) -> (x = y?=w633:bool)
        n348 = Equal?(x="OK", y=w623) -> (x = y?=w631:bool)
        n349 = Select(t=u32 12189624, s=w633, f=u32 16747609) -> (s? t:f=w632:u32)
        n350 = Select(t=u32 12189624, s=w631, f=u32 16747609) -> ()  [unwired: 1 out]
        n351 = property on="Command resp" class="Str"("Text.BGColor"=w632, "Value"=w620) -> ()  [unwired: 2 in, 2 out]
      }
      event "Slave.LO share en": Value Change {
        w665 = "lo_share_enable" ("command")
        n352 = event-data() -> ()  [unwired: 1 in, 6 out]
        n353 = Bundle By Name(cluster=T18 {"Enable"=FALSE} ("Equalization command"), "Enable"="Slave.LO share en") -> (w641:T18)
        n354 = Flatten To JSON(anything=w641) -> (JSON string=w640:string)  [unwired: 2 in, 1 out]
        n355 = call-dynamic "Send Command.vi"("reference in"=w664, "message"=w665, "parameters"=w640, "response?"=TRUE, "timeout"=5000) -> ("status"=w652:string, "reponse"=w649:string, "error out"=w666:errorcluster)  [unwired: 6 in, 2 out]
        n356 = call-dynamic "Send Command.vi"("reference in"=w663, "message"=w665, "parameters"=w640, "response?"=TRUE) -> ("status"=w651:string, "reponse"=w646:string)  [unwired: 7 in, 3 out]
        n357 = call <vilib>:"Flatten To JSON String.vi"("Variant"=w649) -> ("error out"=w647:errorcluster, "JSON String"=w648:string)  [unwired: 9 in]
        n358 = call <vilib>:"Flatten To JSON String.vi"("Variant"=w646) -> ("error out"=w645:errorcluster)  [unwired: 9 in, 1 out]
        n359 = call <vilib>:"Clear Errors.vi"("error in (no error)"=w647) -> ()  [unwired: 5 in, 2 out]
        n360 = call <vilib>:"Clear Errors.vi"("error in (no error)"=w645) -> ()  [unwired: 5 in, 2 out]
        n361 = Equal?(x="OK", y=w652) -> (x = y?=w661:bool)
        n362 = Equal?(x="OK", y=w651) -> (x = y?=w659:bool)
        n363 = Select(t=u32 12189624, s=w661, f=u32 16747609) -> (s? t:f=w660:u32)
        n364 = Select(t=u32 12189624, s=w659, f=u32 16747609) -> ()  [unwired: 1 out]
        n365 = property on="Command resp" class="Str"("Text.BGColor"=w660, "Value"=w648) -> ()  [unwired: 2 in, 2 out]
      }
      event "Analysis.run": Value Change {
        n366 = event-data() -> ()  [unwired: 1 in, 6 out]
        n367 = control-ref of="Analysis"() -> (w667:refnum<vi>)
        n368 = call "GUI process burst data.vi"("Analysis.algo"="Analysis.algo", "TXRX data"=w671, "WaveformGraph in"=w667) -> ("Result param"=w668:string[][], "Result plot"=w669:cluster{"x0":dbl, "dx":dbl, "y":dbl[]}[])  [unwired: 7 in]
        n369 = flat-sequence {
          tunnel: w669 -> [w674]
          tunnel: w668 -> [w673]
          frame #0 {
            # "Analysis done"
            n370 = property on="Analysis res" class="MCListbox (strict)"("ItemNames"=w673) -> ()  [unwired: 2 in, 2 out]
            n371 = local write "Analysis.run"(FALSE) -> ()
            "Analysis" <- w674
          }
        }
      }
      event User Event {
        # "new data arived.\nrefresh available bursts based on group"
        n372 = event-data() -> ("group"=w683:string)  [unwired: 1 in]
        n373 = call "Stall Data Flow.vim"("value in"=w683, "milliseconds to wait"=u32 50) -> ("value out"=w678:string)  [unwired: 1 out]
        n374 = call "DM Get burst list.vi"("burst group"=w678) -> ("error out"=w677:errorcluster, "burst info"=w680:T27)  [unwired: 9 in]
        n375 = Unbundle By Name(w680) -> ("Memory"=w675:dbl, "burst names"=w676:string[])
        n376 = case shown="\"tx\"" w678 {
          tunnel: w676 -> [_ w685 w688]
          tunnel: [_ _ w687] -> w682
          tunnel: w677 -> [_ _ w687]
          tunnel: w675 -> [_ w684 w686]
          frame "False", Default {
          }
          frame "tx" {
            n377 = property on="DM.TX burst list" class="LstBox (strict)"("Item Names"=w685) -> ()  [unwired: 2 in, 2 out]
            "TX records memory" <- w684
          }
          frame "SysA rx", "SysB rx", "rx" {
            n378 = property on="DM.RX burst list" class="LstBox (strict)"("Item Names"=w688) -> ()  [unwired: 2 in, 2 out]
            "RX records memory:" <- w686
          }
        }
      }
      event User Event {
        n379 = event-data() -> ()  [unwired: 1 in, 5 out]
      }
      event User Event {
        n380 = event-data() -> ("error"=w698:T1)  [unwired: 1 in]
        n381 = call "Error cluster to error response.vi"("error in (no error)"=w698, "response"="") -> ("err cluster"=w696:T28)  [unwired: 7 in, 2 out]
        n382 = local read "Error history"() -> (w695:T7)
        n383 = Build Array (concatenate)(w696, w695) -> (w694:T28[])
        n384 = Array Subset(array=w694, length=30) -> (→"Error history":T28[])  [unwired: 1 in]
        n385 = local read "Enable UI"() -> (w691:bool)
        n386 = case shown="True" w691 {
          frame False {
          }
          frame True {
            n387 = local write "Log tab"(enum32{"Command log", "Timing", "Errors"}."Errors" ("Log tab")) -> ()
            n388 = local write "Display tab"(T20."Log" ("Display tab")) -> ()
          }
        }
      }
      event "Log.reset": Value Change {
        n389 = event-data() -> ()  [unwired: 1 in, 6 out]
        n390 = global write "Log GV.vi" "Execution benchmark"(cluster{"command out":T6, "final time":dbl}[] [] ("Execution benchmark")) -> ()
        n391 = local write "Error history"(T7 [] ("Error history")) -> ()
        n392 = global write "Log GV.vi" "Debug log"(string[][] [] ("Debug log")) -> ()
      }
      event "Show all": Value Change {
        n393 = event-data() -> ("NewVal"=w707:bool)  [unwired: 1 in, 5 out]
        n394 = Not(x=w707) -> (.not. x?=w706:bool)
        n395 = property on="command filter" class="Enum (strict)"("Visible"=w706) -> ()  [unwired: 2 in, 2 out]
      }
      event Panel Close? {
        w713 = TRUE
        n396 = event-data() -> ()  [unwired: 1 in, 4 out]
        n397 = global read "Comm GV.vi" "CloseApp"() -> (w712:refnum<user-event>)
        n398 = Generate User Event(user event=w712, event data cluster=TRUE ("event data")) -> (error out=w710:errorcluster)  [unwired: 2 in, 1 out]
        n399 = event-data("Discard?"=w713) -> ()  [unwired: 1 in, 1 out]
      }
      event Menu Selection (App); Menu Selection (User) {
        n400 = event-data() -> ("ItemTag"=w714:string)  [unwired: 1 in, 6 out]
        n401 = case shown="\"Close\"" w714 {
          tunnel: [_ w719] -> w717
          tunnel: [_ TRUE] -> w715
          frame "False", Default {
          }
          frame "Close" {
            n402 = global read "Comm GV.vi" "CloseApp"() -> (w721:refnum<user-event>)
            n403 = Generate User Event(user event=w721, event data cluster=TRUE ("event data")) -> (error out=w719:errorcluster)  [unwired: 2 in, 1 out]
          }
        }
      }
    }
    n404 = local read "Enable UI"() -> (w42:bool)
    n405 = case shown="True" w42 {
      tunnel: w51 -> [_ w54]
      frame False {
      }
      frame True {
        n406 = call <vilib>:"Simple Error Handler.vi"("error in (no error)"=w54) -> ()  [unwired: 4 in, 5 out]
      }
    }
  }
  n407 = while {
    tunnel: w2 -> [_]
    stop <- "stop" stop-if-true
    # "STATUS loop"
    n408 = Wait (ms)(milliseconds to wait=u32 5) -> ()  [unwired: 1 out]
    n409 = global read "HW GV.vi" "HW Status"() -> (→"Instrument status":string)
  }
  n410 = local write "stop"(w3) -> ()
